vi "GUI For test verification.vi"() -> ()   [LabVIEW 2019]
panel:
  out "?":string
  out "?":string
  in  "?":path
  out "?":bool=TRUE
  out "?":bool=TRUE
  out "?":string[][](array[string])
  out "?":string[][](array[string])
  in  "?":string[](array[string])=["a", "b", "f", "g", "h"]
  in  "?":path
  out "?":string[][](array[string])
  out "?":string[][](array[string])
  in  "?":string[](array[string])=["a", "b", "f", "g", "h"]
  # "X AXIS"
  # "FILE  DIRECTORY"
  # "INPUT ARRAY 1"
  # "OUTPUT"
  # "INPUT ARRAY 2"
  # "X AXIS PASS"
  # "Y AXIS  PASS"
  # "Y AXIS"
  # "OUTPUT"
  # "INPUT ARRAY 1"
  # "INPUT ARRAY 2"
  # "FILE DIRECTORY"
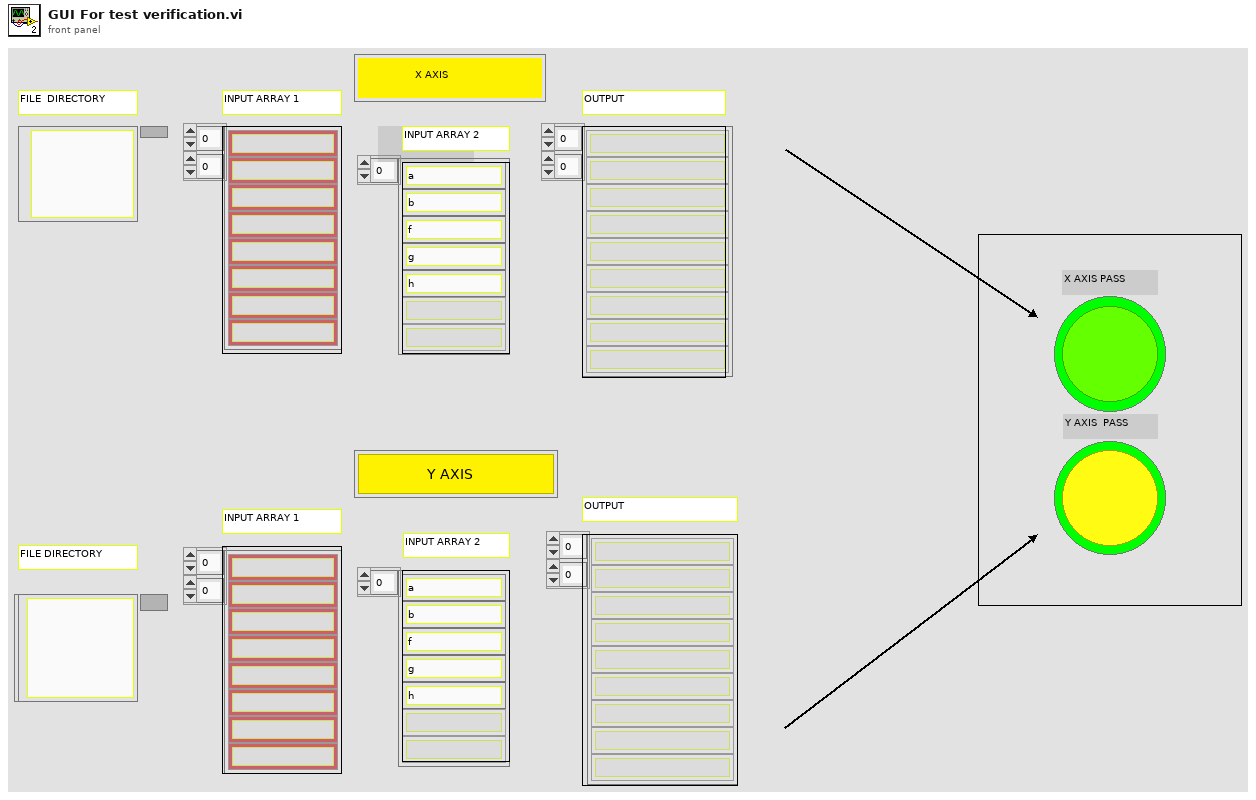
[diagram p1: front panel]
types:
  T1 = enum16{"open", "replace", "create", "open or create", "replace or create", "replace or create with confirmation"}
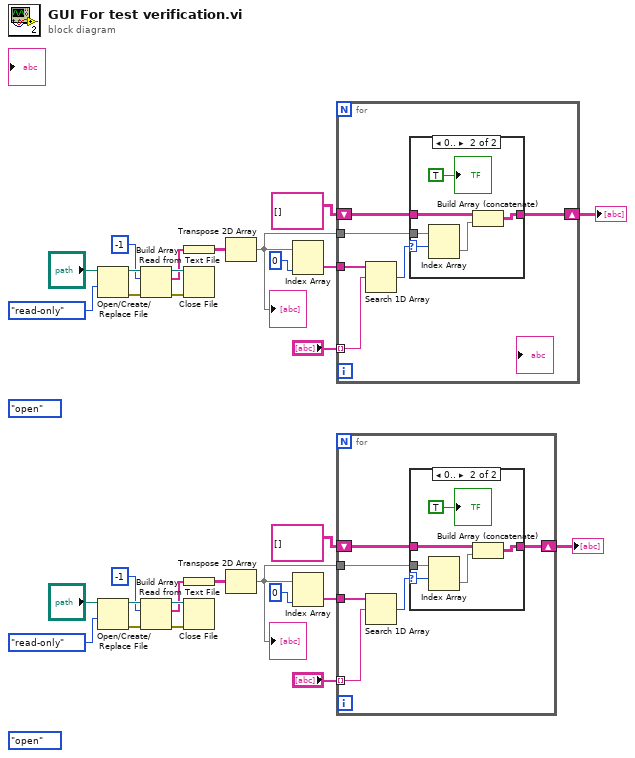
[diagram p0: block diagram]
diagram:
  (unwired) T1."open" ("operation (0:open)")
  (unwired) T1."open" ("operation (0:open)")
  n1 = Open/Create/Replace File(file path (use dialog)="?", access (0:read/write)=enum16{"read/write", "read-only", "write-only"}."read-only") -> (refnum out=w30:refnum<file>, error out=w28:errorcluster)  [unwired: 4 in, 1 out]
  n2 = Open/Create/Replace File(file path (use dialog)="?", access (0:read/write)=enum16{"read/write", "read-only", "write-only"}."read-only") -> (refnum out=w15:refnum<file>, error out=w13:errorcluster)  [unwired: 4 in, 1 out]
  n3 = Read from Text File(file (use dialog)=w30, count=-1, error in=w28) -> (refnum out=w29:refnum<file>, text=w18:string[], error out=w27:errorcluster)  [unwired: 1 in, 1 out]
  n4 = Read from Text File(file (use dialog)=w15, count=-1, error in=w13) -> (refnum out=w14:refnum<file>, text=w3:string[], error out=w12:errorcluster)  [unwired: 1 in, 1 out]
  n5 = Build Array(w18) -> (w19:string[][])
  n6 = Close File(refnum=w29, error in=w27) -> ()  [unwired: 2 out]
  n7 = Build Array(w3) -> (w4:string[][])
  n8 = Close File(refnum=w14, error in=w12) -> ()  [unwired: 2 out]
  n9 = Transpose 2D Array(2D array=w19) -> (transposed array=w17:string[][])
  "?" <- w17
  n10 = Transpose 2D Array(2D array=w4) -> (transposed array=w2:string[][])
  "?" <- w2
  n11 = Index Array(array=w17, index (col)=0 ("disabled index (col)")) -> (element=w22:string[])  [unwired: 1 in]
  n12 = Index Array(array=w2, index (col)=0 ("disabled index (col)")) -> (element=w7:string[])  [unwired: 1 in]
  n13 = for {
    tunnel: "?" -> [w36] mode=indexing
    tunnel: w17 -> [w32]
    tunnel: w22 -> [w35]
    shift-right: [w33] -> w20
    shift-left: string[][] [] -> [w34]
    n14 = Search 1D Array(1D array=w35, element=w36) -> (index of element=w31:i32)  [unwired: 1 in]
    n15 = case shown="0.." w31 {
      selector: w31 -> [_ w39]
      tunnel: w34 -> [w37 w43]
      tunnel: [w37 w42] -> w33
      tunnel: w32 -> [_ w41]
      frame ..-1 {
      }
      frame 0.. {
        n16 = Index Array(array=w41, index (row)=w39) -> (element=w40:string[])  [unwired: 1 in]
        n17 = Build Array (concatenate)(w43, w40) -> (w42:string[][])
        "?" <- TRUE ("ycor  2")
      }
    }
  }
  "?" <- w20
  n18 = for {
    tunnel: "?" -> [w49] mode=indexing
    tunnel: w2 -> [w45]
    tunnel: w7 -> [w48]
    shift-right: [w46] -> w5
    shift-left: string[][] [] -> [w47]
    n19 = Search 1D Array(1D array=w48, element=w49) -> (index of element=w44:i32)  [unwired: 1 in]
    n20 = case shown="0.." w44 {
      selector: w44 -> [_ w52]
      tunnel: w47 -> [w50 w56]
      tunnel: [w50 w55] -> w46
      tunnel: w45 -> [_ w54]
      frame ..-1 {
      }
      frame 0.. {
        n21 = Index Array(array=w54, index (row)=w52) -> (element=w53:string[])  [unwired: 1 in]
        n22 = Build Array (concatenate)(w56, w53) -> (w55:string[][])
        "?" <- TRUE ("ycor  2")
      }
    }
  }
  "?" <- w5
